vi "Write Variable Value.vi"(8 "Error in":errorcluster caption="Error in (no error)", 9 "Response":string, 10 "source/target":string, 11 "Variant Out in":variant) -> (0 "Error out":errorcluster, 3 "Variant Out out":variant)   [LabVIEW 2020, in "CSMStand(Lite).lvlib"]
uses:
  CSMStand(Lite).lvlib
  <userlib>/_NEVSTOP/Communicable State Machine(CSM)/_Shared/CSM Shared.lvlib
  <userlib>/_NEVSTOP/Communicable State Machine(CSM)/Communicable State Machine.lvlib
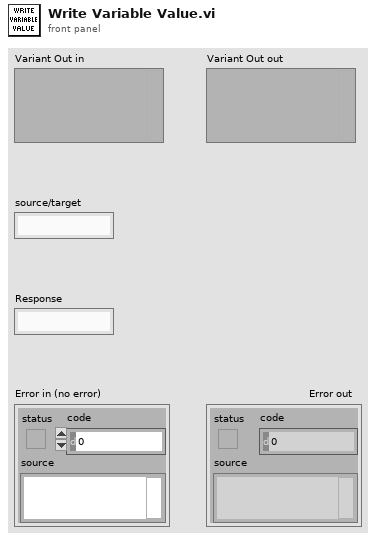
[diagram p1: front panel]
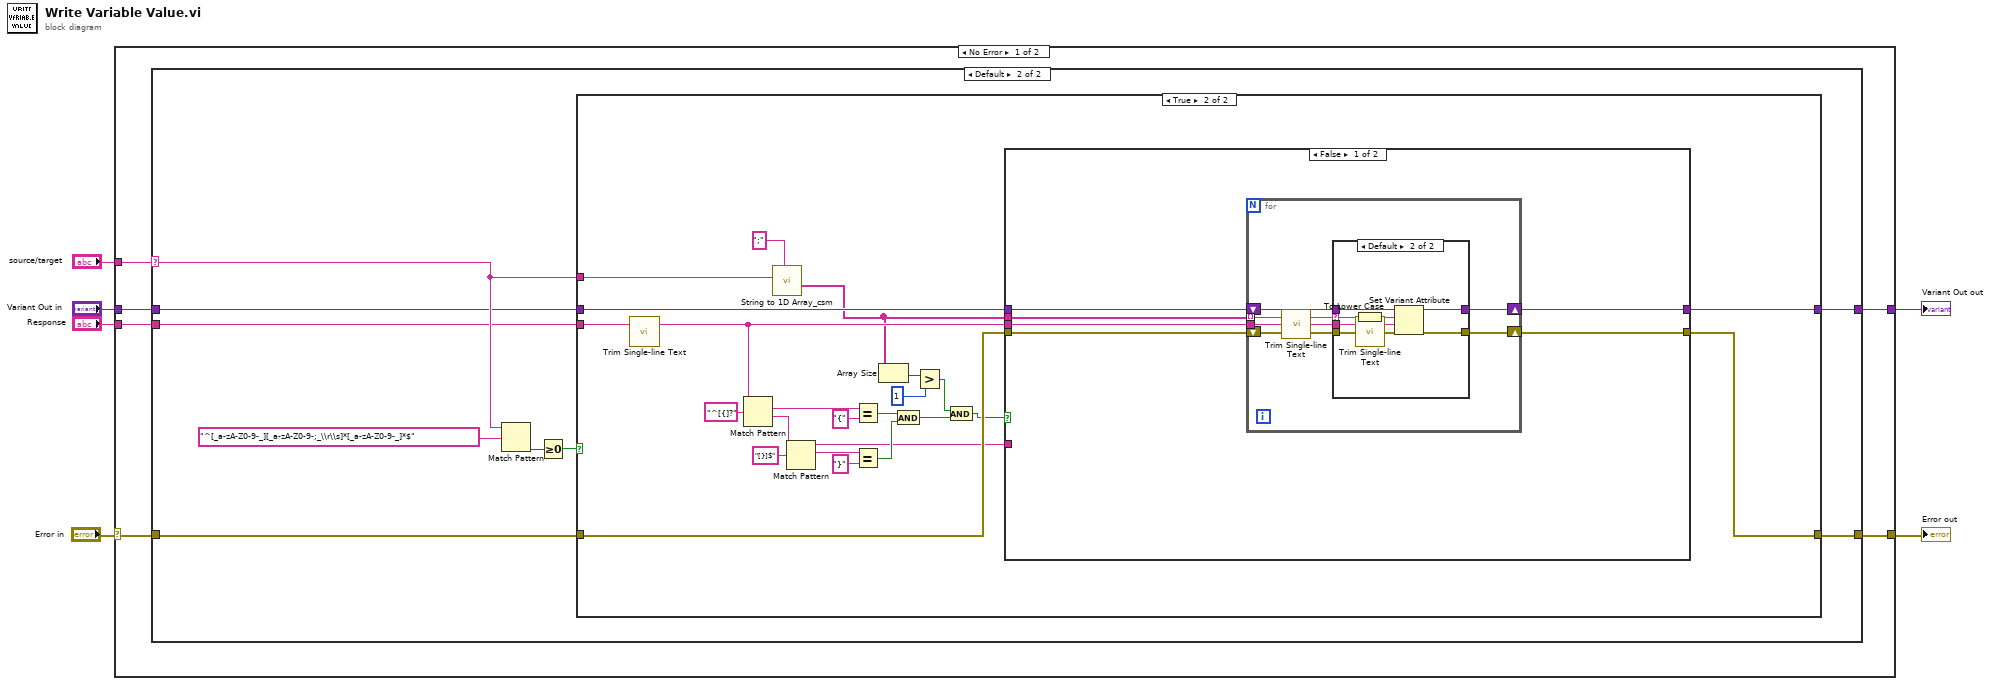
[diagram p0: block diagram]
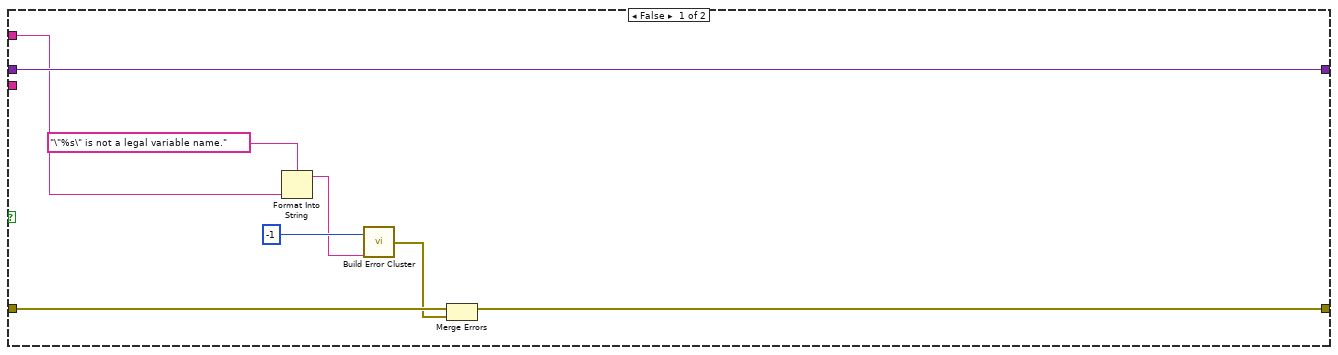
[diagram p3: hidden frame]
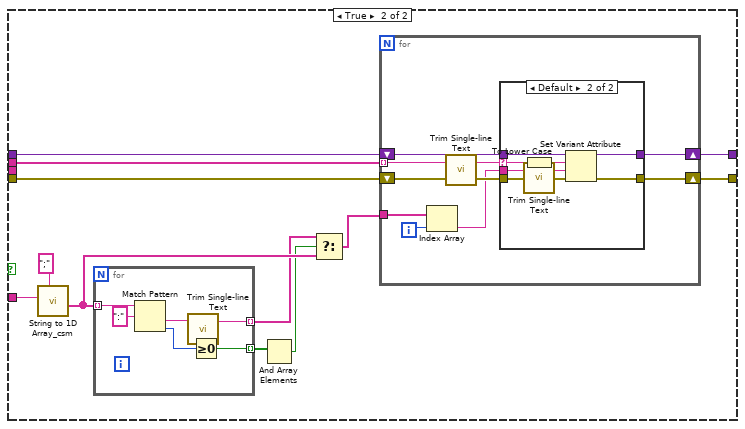
[diagram p5: hidden frame]
diagram:
  n1 = case shown="No Error" "Error in" {
    selector: "Error in" -> [w7 w117]
    tunnel: "source/target" -> [w12 _]
    tunnel: "Response" -> [w11 _]
    tunnel: [w10 w116] -> w4
    tunnel: "Variant Out in" -> [w9 w116]
    tunnel: [w8 w117] -> w2
    frame No Error {
      n2 = case shown="Default" w12 {
        selector: w12 -> [_ w22]
        tunnel: w11 -> [_ w21]
        tunnel: [w14 w20] -> w10
        tunnel: w9 -> [w14 w19]
        tunnel: [w13 w16] -> w8
        tunnel: w7 -> [w13 w15]
        frame "" {
        }
        frame Default {
          n3 = Match Pattern(string=w22, regular expression="^[_a-zA-Z0-9-_][_a-zA-Z0-9-;_\\r\\s]*[_a-zA-Z0-9-_]*$") -> (offset past match=w18:i32)  [unwired: 1 in, 3 out]
          n4 = Greater Or Equal To 0?(x=w18) -> (x >= 0?=w17:bool)
          n5 = case shown="True" w17 {
            tunnel: w22 -> [w25 w49]
            tunnel: w21 -> [_ w51]
            tunnel: [w31 w55] -> w20
            tunnel: w19 -> [w31 w54]
            tunnel: [w28 w53] -> w16
            tunnel: w15 -> [w30 w52]
            frame False {
              n6 = Format Into String(format string="\"%s\" is not a legal variable name.", w25) -> (resulting string=w24:string)  [unwired: 2 in, 1 out]
              n7 = call <userlib>:"Build Error Cluster.vi"("String to Prepend to Source (\"\")"=w24, "Code"=-1) -> ("error out"=w27:errorcluster)
              n8 = Merge Errors(w30, w27) -> (w28:errorcluster)
            }
            frame True {
              n9 = call <userlib>:"Trim Single-line Text.vi"("single-line text"=w51) -> ("trimed text"=w50:string)  [unwired: 2 in]
              n10 = Match Pattern(string=w50, regular expression="^[{]?") -> (match substring=w45:string, after substring=w46:string)  [unwired: 1 in, 2 out]
              n11 = call <userlib>:"String to 1D Array_csm.vi"("delimiter (Tab)"=";", "string"=w49) -> ("Array of Strings"=w36:string[])  [unwired: 9 in]
              n12 = Match Pattern(string=w46, regular expression="[}]$") -> (before substring=w38:string, match substring=w42:string)  [unwired: 1 in, 2 out]
              n13 = Equal?(x=w45, y="{" ("regular expression")) -> (x = y?=w41:bool)
              n14 = Equal?(x=w42, y="}" ("regular expression")) -> (x = y?=w40:bool)
              n15 = Array Size(array=w36) -> (size(s)=w34:i32)
              n16 = And(x=w41, y=w40) -> (x .and. y?=w35:bool)
              n17 = Greater?(x=w34, y=1) -> (0:w32:bool)
              n18 = And(x=w32, y=w35) -> (x .and. y?=w37:bool)
              n19 = case shown="False" w37 {
                tunnel: [w61 w90] -> w55
                tunnel: w54 -> [w60 w89]
                tunnel: [w59 w88] -> w53
                tunnel: w52 -> [w58 w87]
                tunnel: w50 -> [w57 _]
                tunnel: w36 -> [w56 w86]
                tunnel: w38 -> [_ w80]
                frame False {
                  n20 = for {
                    tunnel: w57 -> [w64]
                    tunnel: w56 -> [w63] mode=indexing
                    shift-right: [w68] -> w61
                    shift-left: w60 -> [w67]
                    shift-right: [w66] -> w59
                    shift-left: w58 -> [w65]
                    n21 = call <userlib>:"Trim Single-line Text.vi"("single-line text"=w63) -> ("trimed text"=w62:string)  [unwired: 2 in]
                    n22 = case shown="Default" w62 {
                      selector: w62 -> [_ w76]
                      tunnel: w67 -> [w70 w78]
                      tunnel: [w70 w77] -> w68
                      tunnel: w64 -> [_ w75]
                      tunnel: [w69 w72] -> w66
                      tunnel: w65 -> [w69 w71]
                      frame "" {
                      }
                      frame Default {
                        n23 = To Lower Case(string=w76) -> (all lower case string=w73:string)
                        n24 = call <userlib>:"Trim Single-line Text.vi"("single-line text"=w75) -> ("trimed text"=w74:string)  [unwired: 2 in]
                        n25 = Set Variant Attribute(Variant=w78, name=w73, value=w74, error in=w71) -> (Variant out=w77:variant, error out=w72:errorcluster)  [unwired: 1 out]
                      }
                    }
                  }
                }
                frame True {
                  n26 = call <userlib>:"String to 1D Array_csm.vi"("delimiter (Tab)"=";", "string"=w80) -> ("Array of Strings"=w85:string[])  [unwired: 9 in]
                  n27 = for {
                    tunnel: w85 -> [w93] mode=indexing
                    tunnel: [w92] -> w82 mode=indexing
                    tunnel: [w91] -> w84 mode=indexing
                    n28 = Match Pattern(string=w93, regular expression=":") -> (after substring=w95:string, offset past match=w96:i32)  [unwired: 1 in, 2 out]
                    n29 = call <userlib>:"Trim Single-line Text.vi"("single-line text"=w95) -> ("trimed text"=w91:string)  [unwired: 2 in]
                    n30 = Greater Or Equal To 0?(x=w96) -> (x >= 0?=w92:bool)
                  }
                  n31 = And Array Elements(Boolean array=w82) -> (logical AND=w83:bool)
                  n32 = Select(t=w84, s=w83, f=w85) -> (s? t:f=w79:string[])
                  n33 = for {
                    tunnel: w86 -> [w101] mode=indexing
                    shift-right: [w105] -> w90
                    shift-left: w89 -> [w104]
                    shift-right: [w103] -> w88
                    shift-left: w87 -> [w102]
                    tunnel: w79 -> [w99]
                    i -> [w98]
                    n34 = Index Array(array=w99, index=w98) -> (element=w97:string)
                    n35 = call <userlib>:"Trim Single-line Text.vi"("single-line text"=w101) -> ("trimed text"=w100:string)  [unwired: 2 in]
                    n36 = case shown="Default" w100 {
                      selector: w100 -> [_ w113]
                      tunnel: w104 -> [w107 w115]
                      tunnel: [w107 w114] -> w105
                      tunnel: w97 -> [_ w112]
                      tunnel: [w106 w109] -> w103
                      tunnel: w102 -> [w106 w108]
                      frame "" {
                      }
                      frame Default {
                        n37 = To Lower Case(string=w113) -> (all lower case string=w110:string)
                        n38 = call <userlib>:"Trim Single-line Text.vi"("single-line text"=w112) -> ("trimed text"=w111:string)  [unwired: 2 in]
                        n39 = Set Variant Attribute(Variant=w115, name=w110, value=w111, error in=w108) -> (Variant out=w114:variant, error out=w109:errorcluster)  [unwired: 1 out]
                      }
                    }
                  }
                }
              }
            }
          }
        }
      }
    }
    frame Error {
    }
  }
  "Variant Out out" <- w4
  "Error out" <- w2
